vi "ReplaceCaliperEntry__.vi"(4 "SelectionList":T3[](array[typedef]), 5 "CaliperType":T2 items=["Distance", "Mid Point", "Perpendicular Projection", "Lines Intersection", "Angle from Horizontal", "Angle from Vertical", "Angle Defined by 3 Points", "Angle Defined by 4 Points", "Bissecting Line", "Mid Line", "Center of Mass", "Area", "Line Fit", "Circle Fit", "Ellipse Fit"], 7 "Analysis_Point_Result":T1[](array[typedef]), 10 "CaliperList":i32, 11 "CaliperEntryList":T5[](array[typedef]) {"CaliperType" items=["Distance", "Mid Point", "Perpendicular Projection", "Lines Intersection", "Angle from Horizontal", "Angle from Vertical", "Angle Defined by 3 Points", "Angle Defined by 4 Points", "Bissecting Line", "Mid Line", "Center of Mass", "Area", "Line Fit", "Circle Fit", "Ellipse Fit"]}) -> (3 "CaliperEntryList Out":T5[](array[typedef]) {"CaliperType" items=["Distance", "Mid Point", "Perpendicular Projection", "Lines Intersection", "Angle from Horizontal", "Angle from Vertical", "Angle Defined by 3 Points", "Angle Defined by 4 Points", "Bissecting Line", "Mid Line", "Center of Mass", "Area", "Line Fit", "Circle Fit", "Ellipse Fit"]})   [LabVIEW 2015]
uses:
  Controls/CaliperDataEntry.ctl
  Controls/CaliperType.ctl
  Controls/SelectionListEntry.ctl
  Controls/SelectionListEntryPointType.ctl
  Controls/CaliperResult.ctl
  Analysis/Controls/Analysis_Result_To_Caliper.ctl
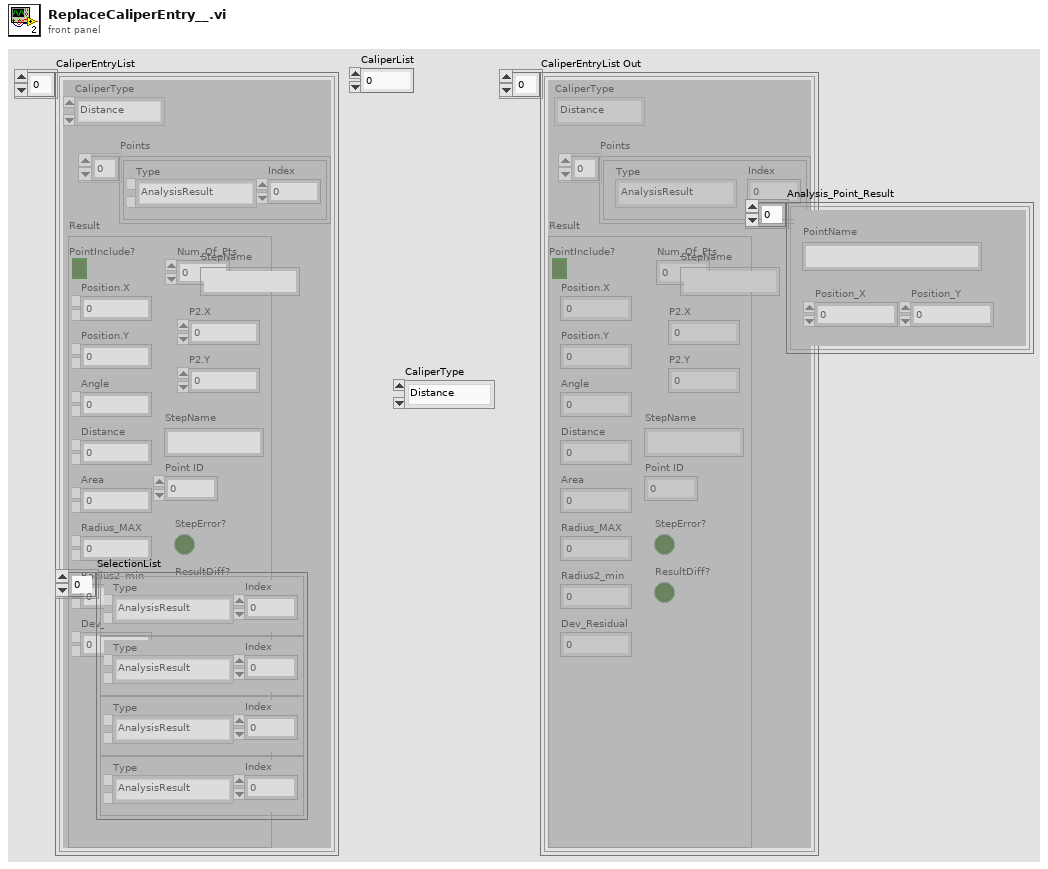
[diagram p1: front panel]
types:
  T1 = typedef "Analysis_Result_To_Caliper.ctl" = cluster{"PointName":string, "Position_X":dbl, "Position_Y":dbl}
  T2 = typedef "CaliperType.ctl" = u32
  T3 = typedef "SelectionListEntry.ctl" = cluster{"Type":T4, "Index":i32}
  T4 = typedef "SelectionListEntryPointType.ctl" = enum16{"AnalysisResult", "CaliperResult"}
  T5 = typedef "CaliperDataEntry.ctl" = cluster{"CaliperType":T2, "Points":T3[], "Result":T6, "StepName":string}
  T6 = typedef "CaliperResult.ctl" = cluster{"PointInclude?":bool, "Num_Of_Pts":u8, "Position.X":dbl, "Position.Y":dbl, "Angle":dbl, "Distance":dbl, "Area":dbl, "Radius_MAX":dbl, "Radius2_min":dbl, "Dev_Residual":dbl, "P2.X":dbl, "P2.Y":dbl, "StepName":string, "Point ID":u8, "StepError?":bool, "ResultDiff?":bool}
  T7 = typedef "CaliperDataEntry_SinglePoint.ctl" = cluster{"CaliperType":T2, "Points":T3[], "Result":T8, "StepName":string}
  T8 = typedef "CaliperResult_SinglePoint.ctl" = cluster{"PointInclude?":bool, "Position.X":dbl, "Position.Y":dbl, "Angle":dbl, "Distance":dbl, "Area":dbl, "Radius_MAX":dbl, "Radius2_min":dbl, "Dev_Residual":dbl, "StepName":string, "Point ID":u8, "StepError?":bool, "ResultDiff?":bool}
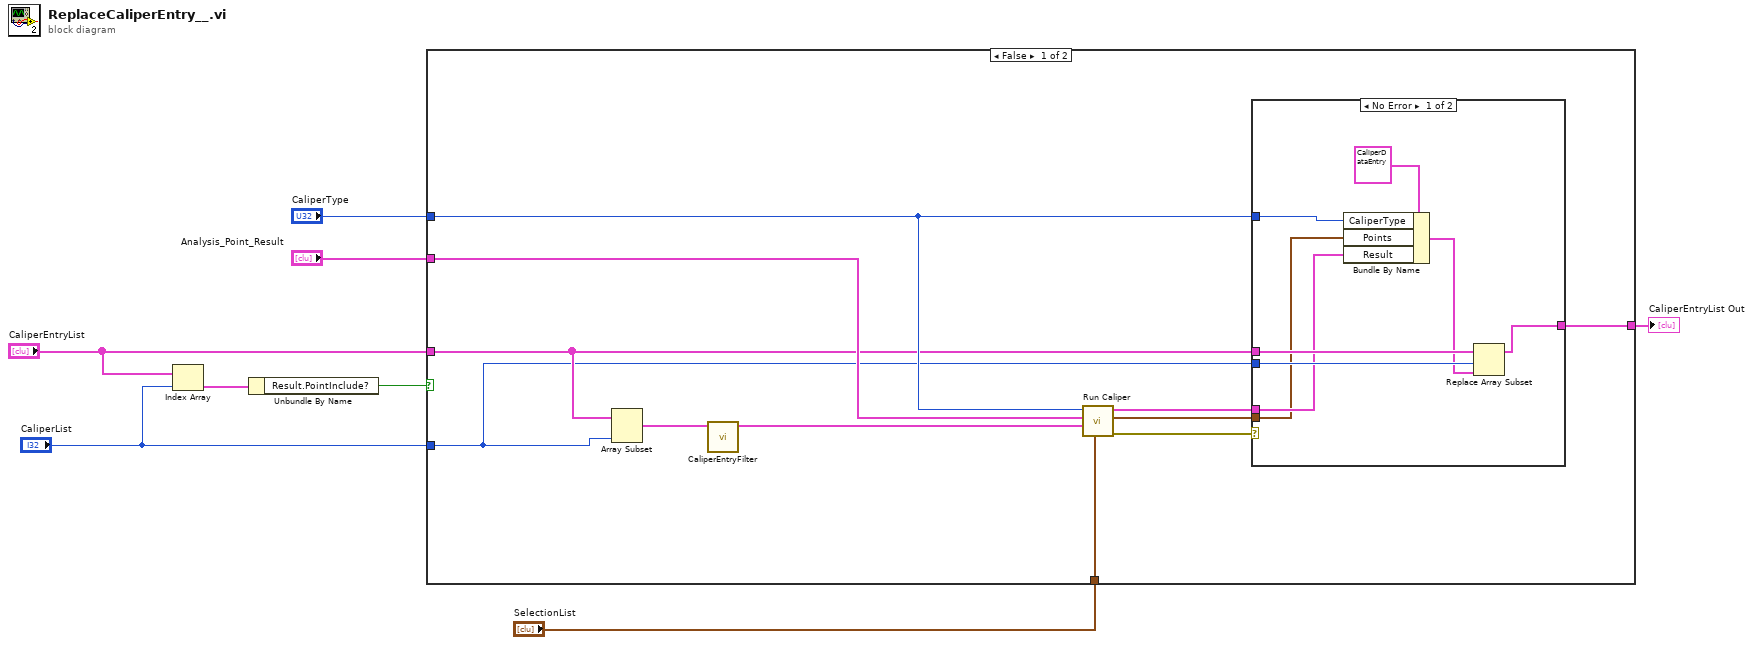
[diagram p0: block diagram]
diagram:
  n1 = Index Array(array="CaliperEntryList", index="CaliperList") -> (element=w7:T5)
  n2 = Unbundle By Name(w7) -> ("Result.PointInclude?"=w6:bool)
  n3 = case shown="False" w6 {
    tunnel: "CaliperEntryList" -> [w12 _]
    tunnel: [w19 _] -> w8
    tunnel: "CaliperList" -> [w10 _]
    tunnel: "CaliperType" -> [w18 _]
    tunnel: "Analysis_Point_Result" -> [w16 _]
    tunnel: "SelectionList" -> [w9 _]
    frame False {
      n4 = Array Subset(array=w12, length=w10) -> (w11:T5[])  [unwired: 1 in]
      n5 = call "CaliperEntryFilter.vi"("CaliperEntryList"=w11) -> ("FilteredCaliperEntry"=w13:T7[])  [unwired: 10 in]
      n6 = call "Run Caliper.vi"("SelectionList"=w9, "FilteredCaliperEntry"=w13, "Analysis_Point_Result"=w16, "CaliperType"=w18) -> ("error out"=w17:errorcluster, "SelectionListOut"=w14:T3[], "Result"=w15:T6)  [unwired: 5 in]
      n7 = case shown="No Error" w17 {
        tunnel: w12 -> [w27 w28]
        tunnel: w10 -> [w26 _]
        tunnel: [w25 w28] -> w19
        tunnel: w18 -> [w23 _]
        tunnel: w15 -> [w21 _]
        tunnel: w14 -> [w20 _]
        frame No Error {
          n8 = Bundle By Name(cluster=T5 {"CaliperType"=0, "Points"=[], "Result"={"PointInclude?"=FALSE, "Num_Of_Pts"=0, "Position.X"=0.0, "Position.Y"=0.0, "Angle"=0.0, "Distance"=0.0, "Area"=0.0, "Radius_MAX"=0.0, "Radius2_min"=0.0, "Dev_Residual"=0.0, "P2.X"=0.0, "P2.Y"=0.0, "StepName"="", "Point ID"=0, "StepError?"=FALSE, "ResultDiff?"=FALSE}, "StepName"=""} ("new element/subarray"), "CaliperType"=w23, "Points"=w20, "Result"=w21) -> (w22:T5)
          n9 = Replace Array Subset(array=w27, new element=w22, index=w26) -> (w25:T5[])
        }
        frame Error {
        }
      }
    }
    frame True {
    }
  }
  "CaliperEntryList Out" <- w8
